vi "LInsert.vi"(0 "reference in":refnum<class "Redis.lvclass">, 1 "Key":string, 5 "Pivot":string, 9 "Value":string, 11 "Error In":errorcluster, 12 "Order":enum16{"Before", "After"}(ring)) -> (4 "reference out":refnum<class "Redis.lvclass">, 8 "Data":T1, 15 "Error Out":errorcluster)   [LabVIEW 2020, in "Redis.lvclass"]
doc: "<b>LINSERT</b>\n\nInserts element in the list stored at key either before or after the reference value pivot.\n\nWhen key does not exist, it is considered an empty list and no operation is performed.\n\nAn error is returned when key exists but does not hold a list value."
uses:
  Redis.lvclass
  ReplyDataTypeEnum.ctl
  RedisDataType.ctl
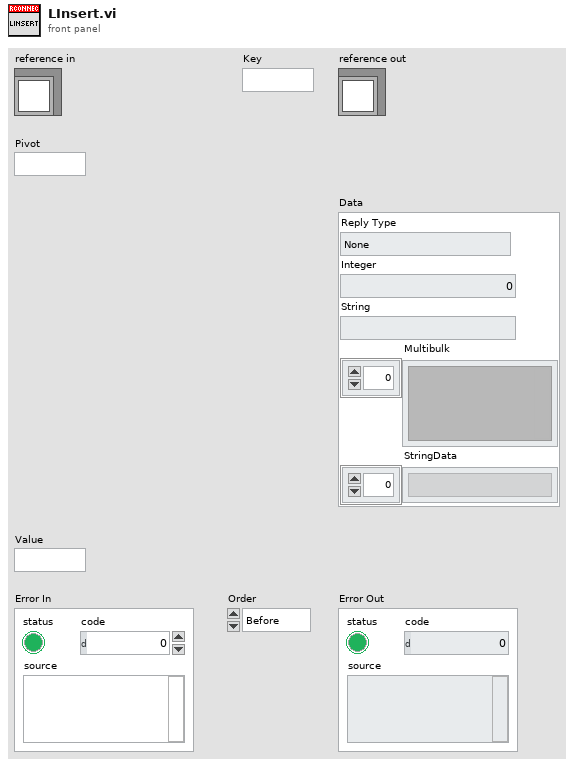
[diagram p1: front panel]
types:
  T1 = typedef "Redis.lvclass/RedisDataType.ctl" = cluster{"Reply Type":T2, "Integer":i64, "String":string, "Multibulk":variant[], "StringData":string[]}
  T2 = typedef "Redis.lvclass/ReplyDataTypeEnum.ctl" = enum16{"None", "Error", "Status", "Nil", "Integer", "String", "Multibulk"}
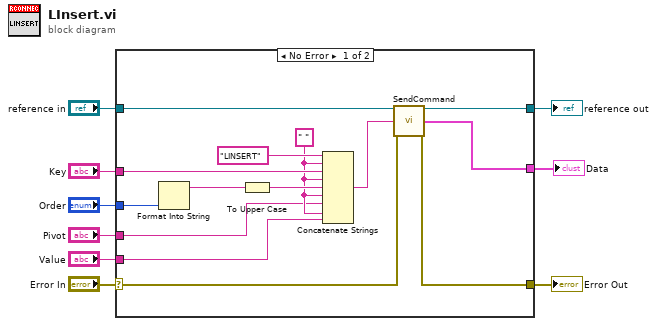
[diagram p0: block diagram]
diagram:
  n1 = case shown="No Error" "Error In" {
    selector: "Error In" -> [w21 w25]
    tunnel: [w20 w25] -> w8
    tunnel: [w23 w24] -> w6
    tunnel: "reference in" -> [w22 w24]
    tunnel: [w19 _] -> w5
    tunnel: "Key" -> [w17 _]
    tunnel: "Order" -> [w15 _]
    tunnel: "Pivot" -> [w11 _]
    tunnel: "Value" -> [w10 _]
    frame No Error {
      w12 = " "
      n2 = Format Into String(w15) -> (resulting string=w14:string)  [unwired: 3 in, 1 out]
      n3 = To Upper Case(1:w14) -> (0:w13:string)
      n4 = Concatenate Strings("LINSERT", w12, w17, w12, w13, w12, w11, w12, w10) -> (w16:string)
      n5 = call "SendCommand.vi"("reference in"=w22, "Command"=w16, "Error In"=w21) -> ("reference out"=w23:refnum<class "Redis.lvclass">, "Data"=w19:T1, "Error Out"=w20:errorcluster)  [unwired: 10 in]
    }
    frame Error {
    }
  }
  "Error Out" <- w8
  "reference out" <- w6
  "Data" <- w5
